vi "1 button.vi"(3 "error in":errorcluster, 5 "Pop-up Input":T1) -> (0 "error out":errorcluster, 1 "Pressed Button":string, 2 "Message":string)   [LabVIEW 2019, in "ZenGage v3.0 UI.lvclass"]
uses:
  ZenGage v3.0 UI.lvclass
  Common/Controls/Pop-up Input.ctl
panel:
  in  "SoftwareExit_Inspection":bool
  in  "Button 2":bool
  out "Title Display":string="Confirmation STATUS......"
  out "Message Display":string="LOGIN STATUS......"
  in  "Button 1":bool
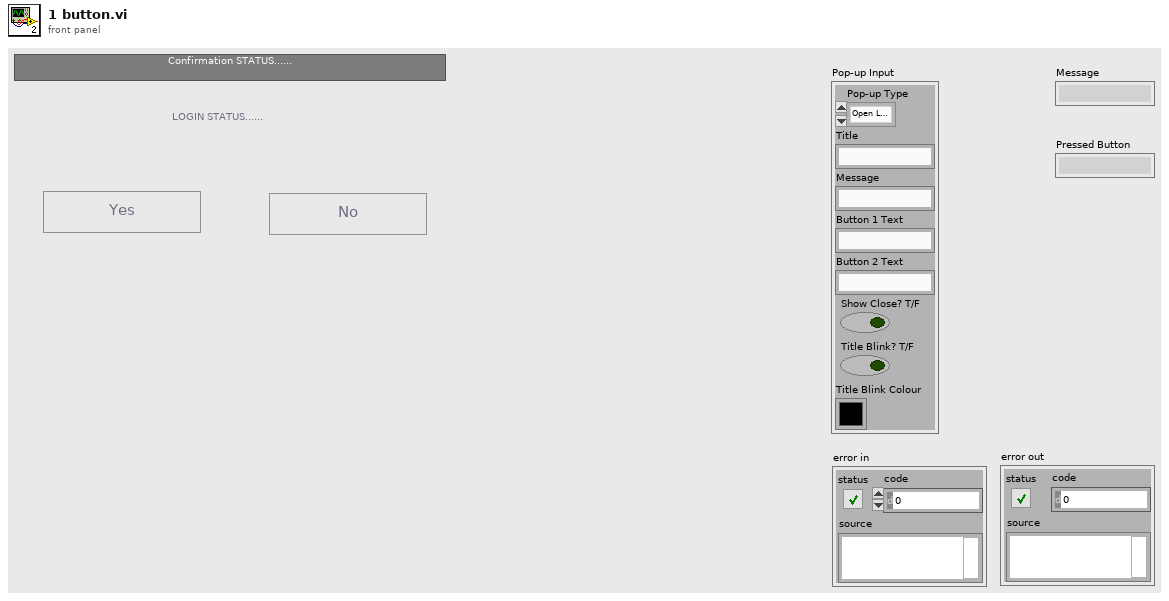
[diagram p1: front panel]
types:
  T1 = typedef "Pop-up Input.ctl" = cluster{"Pop-up Type":enum16{"Open Logo Display", "Close Logo Display", "Open Loading Bar", "Close Loading Bar", "Open Alert Display", "Close Alert Display", "One button dialog box", "Two button dialog box", "User Authentication"}, "Title":string, "Message":string, "Button 1 Text":string, "Button 2 Text":string, "Show Close? T/F":bool, "Title Blink? T/F":bool, "Title Blink Colour":u32}
  T2 = cluster{"Default Title Text Colour":u32, "Default Message Text Colour":u32, "Default Button 1 Text Colour":u32, "Default Button 2 Text Colour":u32, "Tile Text.Font:Bold":bool, "Message Text.Font:Bold":bool, "Button 1 Text.Font:Bold":bool, "Button 2 Text.Font:Bold":bool, "Close Button Text.Font:Bold":bool, "Title Text Size":u64, "Message Text size":u64, "Button1 & Button2 Text Size":u64, "Close Text Size":u64}
  T3 = enum16{"Open Logo Display", "Close Logo Display", "Open Loading Bar", "Close Loading Bar", "Open Alert Display", "Close Alert Display", "One button dialog box", "Two button dialog box", "User Authentication"}
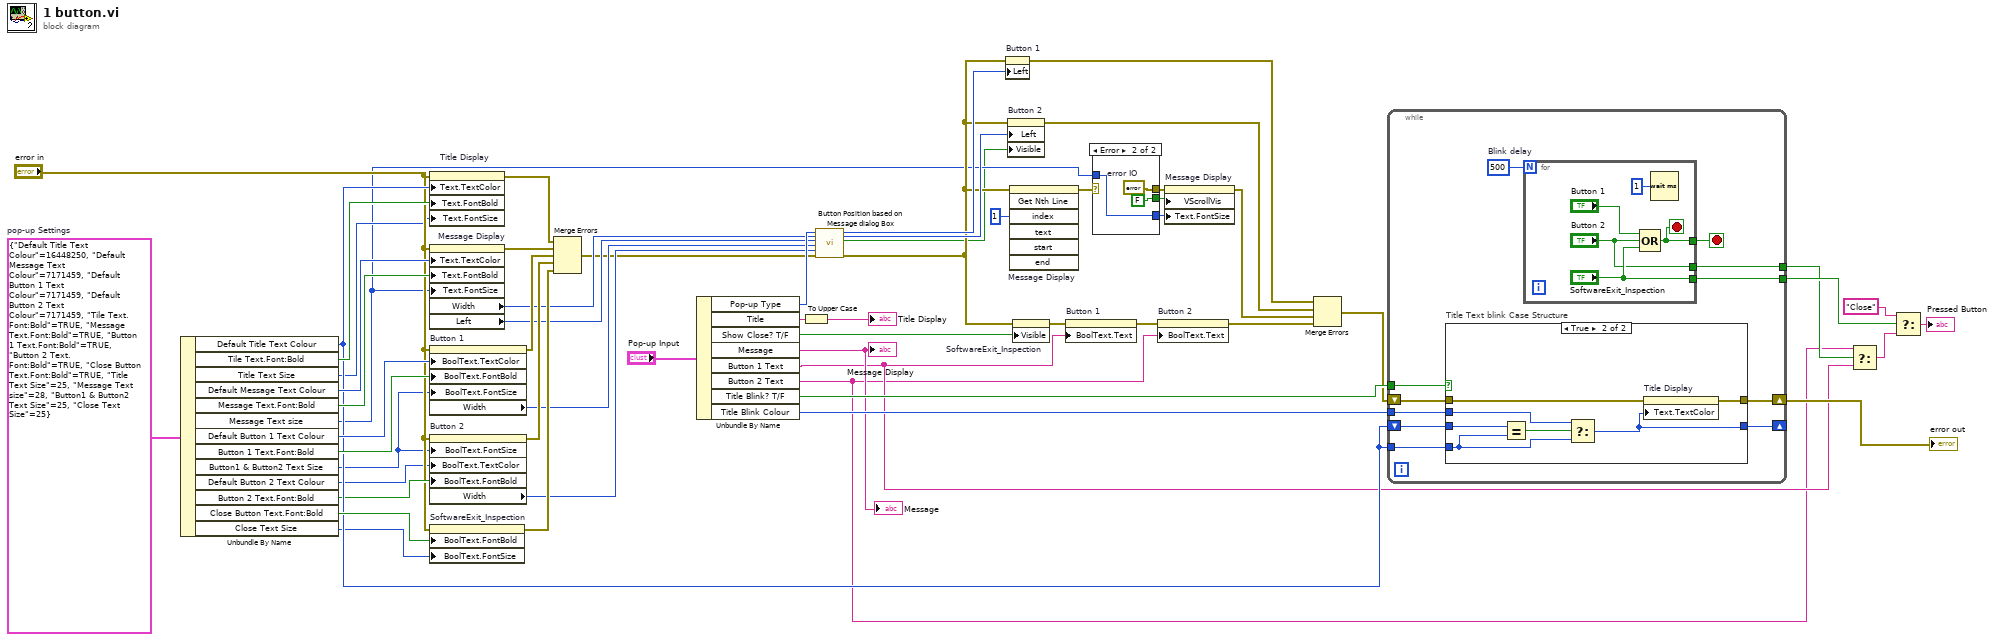
[diagram p0: block diagram]
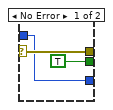
[diagram p2: hidden frame]
diagram:
  w50 = T2 {"Default Title Text Colour"=16448250, "Default Message Text Colour"=7171459, "Default Button 1 Text Colour"=7171459, "Default Button 2 Text Colour"=7171459, "Tile Text.Font:Bold"=TRUE, "Message Text.Font:Bold"=TRUE, "Button 1 Text.Font:Bold"=TRUE, "Button 2 Text.Font:Bold"=TRUE, "Close Button Text.Font:Bold"=TRUE, "Title Text Size"=25, "Message Text size"=28, "Button1 & Button2 Text Size"=25, "Close Text Size"=25}  # pop-up Settings
  n1 = Unbundle By Name(w50) -> ("Default Title Text Colour"=w39:u32, "Tile Text.Font:Bold"=w48:bool, "Title Text Size"=w28:u64, "Default Message Text Colour"=w47:u32, "Message Text.Font:Bold"=w46:bool, "Message Text size"=w5:u64, "Default Button 1 Text Colour"=w45:u32, "Button 1 Text.Font:Bold"=w44:bool, "Button1 & Button2 Text Size"=w7:u64, "Default Button 2 Text Colour"=w8:u32, "Button 2 Text.Font:Bold"=w38:bool, "Close Button Text.Font:Bold"=w49:bool, "Close Text Size"=w6:u64)
  n2 = property on="Title Display" class="Str"(error in="error in", "Text.TextColor"=w39, "Text.FontBold"=w48, "Text.FontSize"=w28) -> (error out=w43:errorcluster)  [unwired: 1 in, 1 out]
  n3 = property on="Message Display" class="Str"(error in="error in", "Text.TextColor"=w47, "Text.FontBold"=w46, "Text.FontSize"=w5) -> (error out=w42:errorcluster, "Width"=w21:u32, "Left"=w20:i32)  [unwired: 1 in, 1 out]
  n4 = property on="Button 1" class="Bool"(error in="error in", "BoolText.TextColor"=w45, "BoolText.FontBold"=w44, "BoolText.FontSize"=w7) -> (error out=w41:errorcluster, "Width"=w19:u32)  [unwired: 1 in, 1 out]
  n5 = property on="Button 2" class="Bool"(error in="error in", "BoolText.FontSize"=w7, "BoolText.TextColor"=w8, "BoolText.FontBold"=w38) -> (error out=w36:errorcluster, "Width"=w18:u32)  [unwired: 1 in, 1 out]
  n6 = property on="SoftwareExit_Inspection" class="Bool (strict)"(error in="error in", "BoolText.FontBold"=w49, "BoolText.FontSize"=w6) -> (error out=w40:errorcluster)  [unwired: 1 in, 1 out]
  n7 = Merge Errors(w43, w42, w41, w36, w40) -> (w17:errorcluster)
  n8 = Unbundle By Name("Pop-up Input") -> ("Pop-up Type"=w32:T3, "Title"=w56:string, "Show Close? T/F"=w24:bool, "Message"=→"Message" →"Message Display":string, "Button 1 Text"=w2:string, "Button 2 Text"=w1:string, "Title Blink? T/F"=w52:bool, "Title Blink Colour"=w51:u32)
  n9 = To Upper Case(1:w56) -> (0:→"Title Display":string)
  n10 = call "Button Position based on Message dialog Box.vi"("Pop-up Type"=w32, "Message Width"=w21, "Message Left"=w20, "Button 1 Width"=w19, "Button 2 Width"=w18, "error in (no error)"=w17) -> ("Button 1 Left"=w30:u32, "Button 2 Left"=w31:u32, "Button Visible"=w3:bool, "error out"=w15:errorcluster)  [unwired: 10 in]
  n11 = property on="Button 1" class="Bool"(error in=w15, "Left"=w30) -> (error out=w10:errorcluster)  [unwired: 1 in, 1 out]
  n12 = property on="Button 2" class="Bool"(error in=w15, "Left"=w31, "Visible"=w3) -> (error out=w11:errorcluster)  [unwired: 1 in, 1 out]
  n13 = invoke on="Message Display" class="Str" method="Get Nth Line"(error in=w15, "index"=u32 1 ("line index")) -> (error out=w26:errorcluster)  [unwired: 5 in, 6 out]
  n14 = property on="SoftwareExit_Inspection" class="Bool (strict)"(error in=w15, "Visible"=w24) -> (error out=w14:errorcluster)  [unwired: 1 in, 1 out]
  n15 = property on="Button 1" class="Bool"(error in=w14, "BoolText.Text"=w2) -> (error out=w16:errorcluster)  [unwired: 1 in, 1 out]
  n16 = case shown="Error" w26 {
    selector: w26 -> [w60 _]
    tunnel: [w60 w63] -> w22
    tunnel: [TRUE ("Horizontal Scrollbar Visible") FALSE ("Horizontal Scrollbar Visible")] -> w27
    tunnel: w5 -> [w58 w61]
    tunnel: [w58 w61] -> w4
    frame No Error {
    }
    frame Error {
      w63 = errorcluster {"status"=FALSE, "code"=0, "source"=""}  # error IO
    }
  }
  n17 = property on="Button 2" class="Bool"(error in=w16, "BoolText.Text"=w1) -> (error out=w13:errorcluster)  [unwired: 1 in, 1 out]
  n18 = property on="Message Display" class="Str"(error in=w22, "VScrollVis"=w27, "Text.FontSize"=w4) -> (error out=w12:errorcluster)  [unwired: 1 in, 1 out]
  n19 = Merge Errors(w10, w11, w12, w13) -> (w9:errorcluster)
  n20 = while {
    shift-right: [w65] -> w53
    shift-left: w9 -> [w69]
    tunnel: [w74] -> w35
    tunnel: w52 -> [w73]
    shift-right: [w70] -> _
    shift-left: w39 -> [w72]
    tunnel: w51 -> [w71]
    tunnel: w39 -> [w68]
    tunnel: [w67] -> w33
    stop <- w64 stop-if-true
    w66 = 500  # Blink delay
    n21 = case "Title Text blink Case Structure" shown="True" w73 {
      tunnel: w69 -> [w80 w88]
      tunnel: w72 -> [_ w87]
      tunnel: w71 -> [_ w82]
      tunnel: [w81 w85] -> w70
      tunnel: w68 -> [w81 w84]
      tunnel: [w80 w83] -> w65
      frame False {
      }
      frame True {
        n22 = Equal?(x=w87, y=w84) -> (x = y?=w86:bool)
        n23 = Select(t=w82, s=w86, f=w84) -> (s? t:f=w85:u32)
        n24 = property on="Title Display" class="Str"(error in=w88, "Text.TextColor"=w85) -> (error out=w83:errorcluster)  [unwired: 1 in, 1 out]
      }
    }
    n25 = for {
      N: w66 -> [_]
      tunnel: [w76] -> w64
      tunnel: ["SoftwareExit_Inspection"] -> w74
      tunnel: ["Button 2"] -> w67
      stop <- w76 stop-if-true
      n26 = Compound Arithmetic op=OR("Button 1", "Button 2", "SoftwareExit_Inspection") -> (w76:bool)
      n27 = Wait (ms)(milliseconds to wait=u32 1) -> ()  [unwired: 1 out]
    }
  }
  "error out" <- w53
  n28 = Select(t=w1, s=w33, f=w2) -> (s? t:f=w34:string)
  n29 = Select(t="Close", s=w35, f=w34) -> (s? t:f=→"Pressed Button":string)
